vi "Obtain Unique ID.vi"(11 "IObserver In":refnum<class "IObserver.lvclass">) -> (0 "error out":errorcluster, 3 "IObserver Out":refnum<class "IObserver.lvclass">)   [LabVIEW 2017, in "IObserver.lvlib" / "IObserver.lvclass"]
doc: "<License>\nCopyright © 2017 Composed Systems, LLC | All rights reserved\nwww.composed.io\n\nAuthor: Ethan Stern <ethan.stern@composed.io>\n\nThis software is provided \"AS IS\" WITHOUT WARRANTIES, either express or implied, AND IS FOR EDUCATIONAL PURPOSES ONLY.\n</License>"
uses:
  IObserver.lvclass
  C:/Program Files (x86)/National Instruments/LabVIEW 2017/vi.lib/ActorFramework/Actor/Actor.lvclass
  <vilib>/ActorFramework/Actor/Actor.lvclass/Actor.ctl
  <vilib>/ActorFramework/Message Enqueuer/Message Enqueuer.lvclass/Message Enqueuer.ctl
  IObserver.lvclass/IObserver.ctl
  <vilib>/ActorFramework/Message Enqueuer/Init from Existing Queue.vi
  <vilib>/Utility/error.llb/Error Cluster From Error Code.vi
  <vilib>/ErrorRing/Error Ring.xnode
  <vilib>/ActorFramework/Message Enqueuer/Message Enqueuer.lvclass
  <vilib>/ActorFramework/Actor/Actor.lvclass
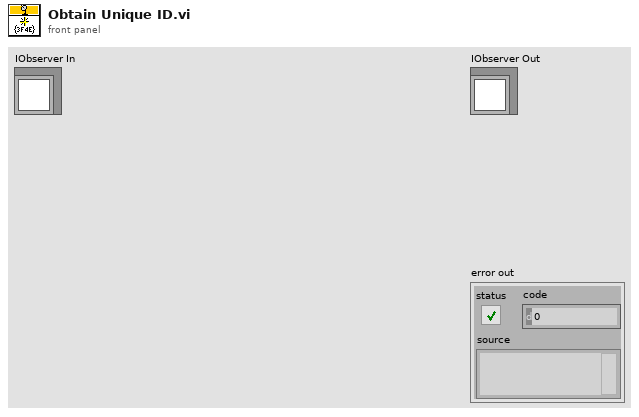
[diagram p1: front panel]
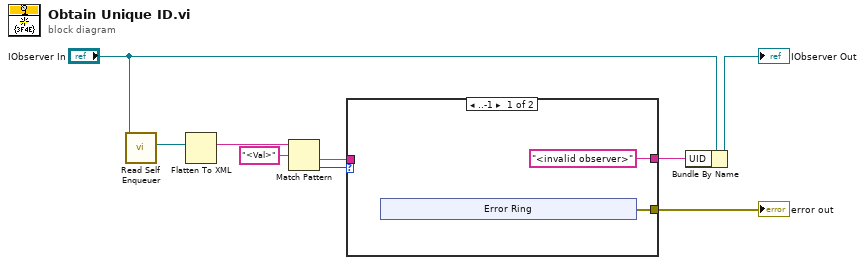
[diagram p0: block diagram]
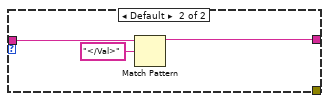
[diagram p2: hidden frame]
diagram:
  n1 = call <vilib>:"Read Self Enqueuer.vi"("Actor"="IObserver In") -> ("Self Enqueuer"=w5:refnum<class "Message Enqueuer.lvclass">)  [unwired: 10 in]
  n2 = Flatten To XML(anything=w5) -> (xml string=w7:string)
  n3 = Match Pattern(string=w7, regular expression="<Val>") -> (after substring=w8:string, offset past match=w9:i32)  [unwired: 1 in, 2 out]
  n4 = case shown="..-1" w9 {
    tunnel: w8 -> [_ w19]
    tunnel: ["<invalid observer>" ("xml string") w17] -> w2
    tunnel: [w10 _] -> w1
    frame ..-1 {
      n5 = xnode "Error Ring"() -> ("error out"=w10:errorcluster)
    }
    frame Default {
      n6 = Match Pattern(string=w19, regular expression="</Val>") -> (before substring=w17:string)  [unwired: 1 in, 3 out]
    }
  }
  "error out" <- w1
  n7 = Bundle By Name(cluster="IObserver In", "UID"=w2) -> (→"IObserver Out":refnum<class "IObserver.lvclass">)
